vi "YAML.List.vi"(2 "Key":string, 3 "lines":string[](array[string])) -> (1 "Output":string)   [LabVIEW 2016, in "AFM Control.lvclass"]
uses:
  AFM Control.lvclass
panel:
  # "This entire block of text will be the value of the 'literal_block' key,\n    with line breaks being preserved.\n\n    The literal continues until de-dented, and the leading indentation is\n    stripped.\n\n        Any lines that are 'more-indented' keep the rest of their indentation -\n        these lines will be indented by 4 spaces."
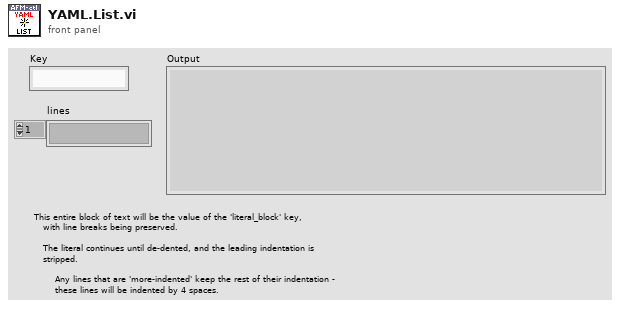
[diagram p1: front panel]
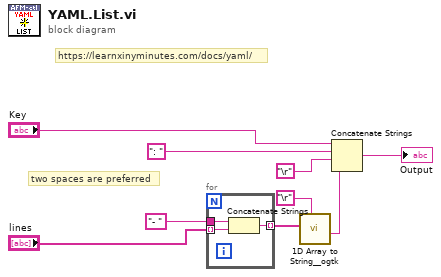
[diagram p0: block diagram]
diagram:
  # "two spaces are preferred"
  # "https://learnxinyminutes.com/docs/yaml/"
  n1 = for {
    tunnel: "lines" -> [w12] mode=indexing
    tunnel: "- " ("string") -> [w10]
    tunnel: [w11] -> w5 mode=indexing
    n2 = Concatenate Strings(w10, w12) -> (w11:string)
  }
  n3 = call <userlib>:"1D Array to String__ogtk.vi"("delimiter (Tab)"="\r", "Array of Strings"=w5) -> ("delimited string"=w7:string)  [unwired: 9 in]
  n4 = Concatenate Strings("Key", ": " ("string"), "\r", w7) -> (→"Output":string)
